vi "linkam.getTemp2.vi"(8 "error in (no error)":errorcluster, 11 "VISA resource name in":refnum<visa-resource-name>) -> (0 "error out":errorcluster, 2 "temp":dbl format="%.2g", 3 "VISA resource name out":refnum<visa-resource-name>)   [LabVIEW 8.6]
panel:
  out "read buffer":string
  out "return count 2":u32
  out "return count":u32
  out "substring":string
  in  "Serial Settings:Number of Bytes at Serial Port":u32
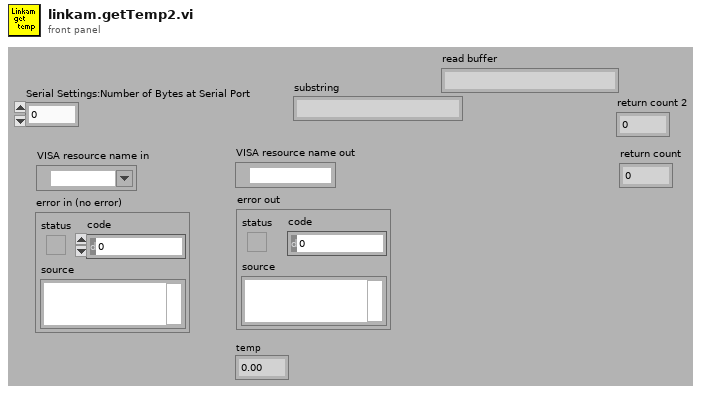
[diagram p1: front panel]
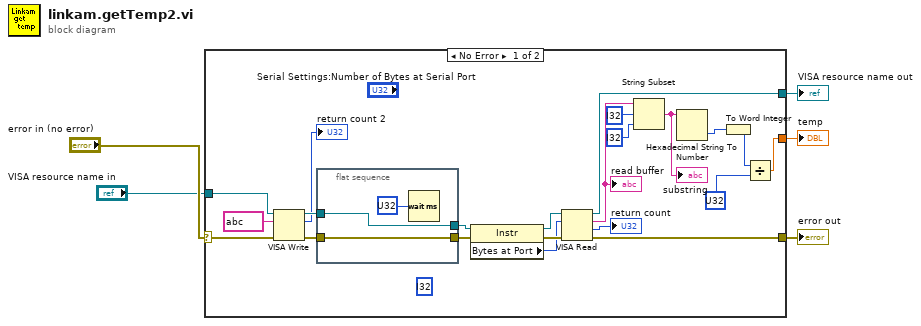
[diagram p0: block diagram]
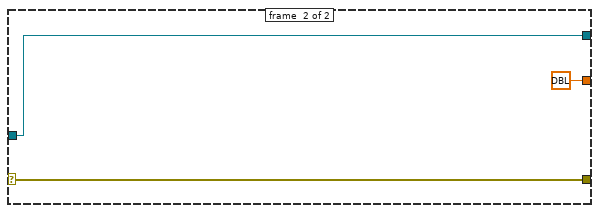
[diagram p2: hidden frame]
diagram:
  n1 = case shown="No Error" "error in (no error)" {
    selector: "error in (no error)" -> [w27 w33]
    tunnel: [w26 w33] -> w4
    tunnel: [w25 w31] -> w5
    tunnel: [w17 dbl ?] -> w3
    tunnel: "VISA resource name in" -> [w8 w31]
    frame #0 {
      (unwired) i32 ? ("length (rest)")
      n2 = VISA Write(VISA resource name=w8, write buffer=string ? ("String"), error in (no error)=w27) -> (VISA resource name out=w20:refnum<visa-resource-name>, return count=→"return count 2":u32, error out=w21:errorcluster)
      n3 = flat-sequence {
        tunnel: [w28] -> w14
        tunnel: w21 -> [w29]
        tunnel: [w29] -> w12
        tunnel: w20 -> [w28]
        frame #0 {
          n4 = Wait (ms)(milliseconds to wait=u32 ?) -> ()  [unwired: 1 out]
        }
      }
      n5 = property class="Instr"(reference=w14, error in=w12) -> (reference out=w13:refnum<visa-resource-name>, error out=w11:errorcluster, "Bytes at Port"=w10:u32)
      n6 = VISA Read(VISA resource name=w13, byte count=w10, error in (no error)=w11) -> (VISA resource name out=w25:refnum<visa-resource-name>, read buffer=w19:string, return count=→"return count":u32, error out=w26:errorcluster)
      "read buffer" <- w19
      n7 = String Subset(string=w19, offset (0)=i32 ?, length (rest)=i32 ? ("length (rest)")) -> (substring=w22:string)
      "substring" <- w22
      n8 = Hexadecimal String To Number(string=w22) -> (number=w7:u32)  [unwired: 2 in, 1 out]
      n9 = To Word Integer(number=w7) -> (16bit integer=w6:i16)
      n10 = Divide(x=w6, y=u32 ?) -> (x/y=w17:dbl)
    }
    frame #1 {
    }
  }
  "VISA resource name out" <- w5
  "error out" <- w4
  "temp" <- w3
